vi "Get Output Values.vi"(6 "Last request":bool, 8 "error in (no error)":errorcluster, 10 "Number of points":i32, 11 "Spectrum Recorder in":refnum<class "Spectrum Recorder too.lvclass">) -> (0 "error out":errorcluster, 2 "Output values":dbl[](array[numeric]), 3 "Spectrum Recorder out":refnum<class "Spectrum Recorder too.lvclass">)   [LabVIEW 2016, in "Spectrum Recorder too.lvclass"]
uses:
  Spectrum Recorder too.lvclass
  C:/github/LabActor/Instrument Actor/Instrument Actor.lvclass
  Spectrum Recorder too.lvclass/Spectrum Recorder too.ctl
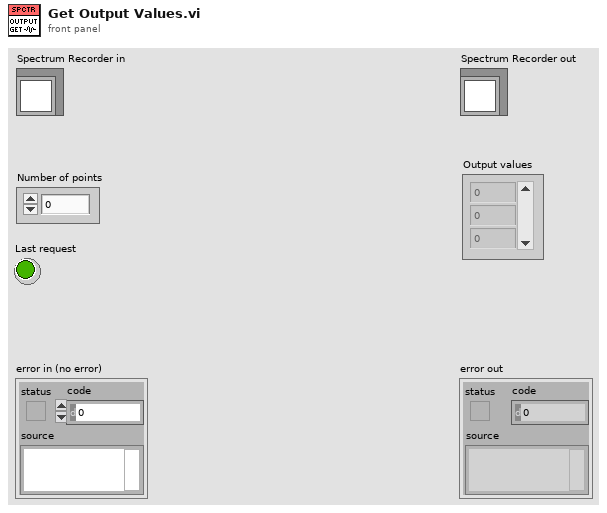
[diagram p1: front panel]
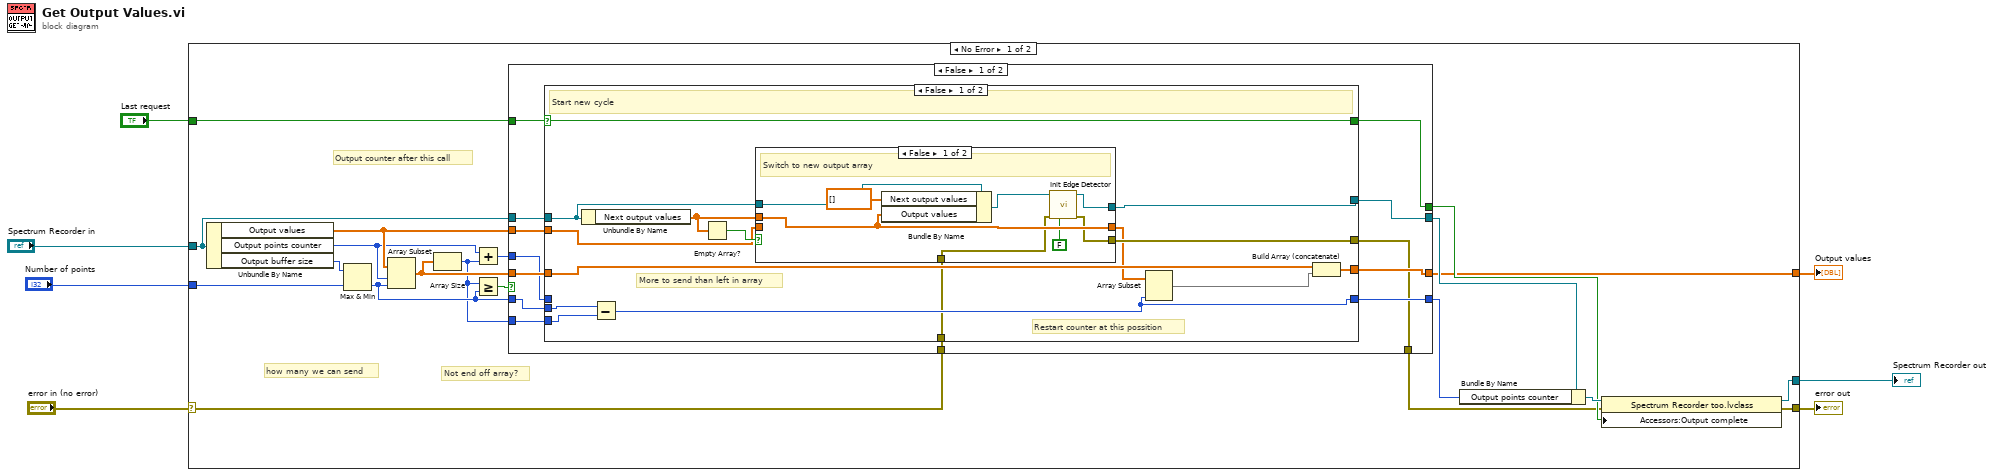
[diagram p0: block diagram]
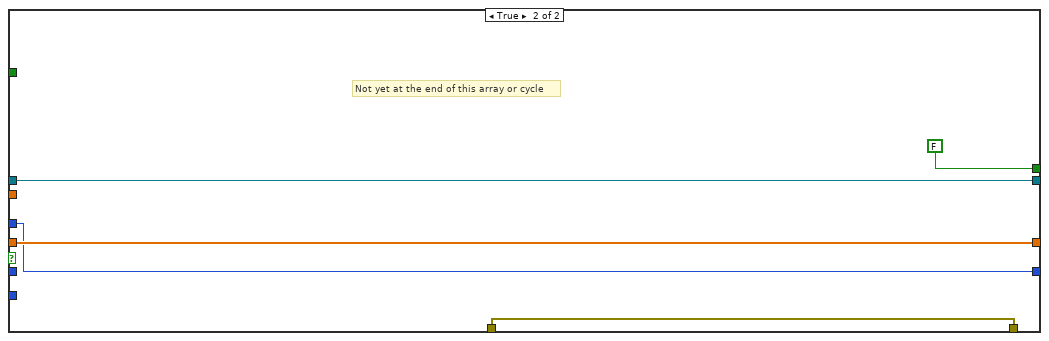
[diagram p4: hidden frame]
diagram:
  n1 = case shown="No Error" "error in (no error)" {
    selector: "error in (no error)" -> [w11 w78]
    tunnel: [w27 w78] -> w6
    tunnel: [w25 w77] -> w4
    tunnel: "Spectrum Recorder in" -> [w22 w77]
    tunnel: "Number of points" -> [w15 _]
    tunnel: [w10 _] -> w2
    tunnel: "Last request" -> [w23 _]
    frame No Error {
      # "Not end off array?"
      # "Output counter after this call"
      # "how many we can send"
      n2 = Unbundle By Name(w22) -> ("Output values"=w20:dbl[], "Output points counter"=w9:i32, "Output buffer size"=w14:i32)
      n3 = Max & Min(x=w14, y=w15) -> (min(x,y)=w21:i32)  [unwired: 1 out]
      n4 = Array Subset(array=w20, index=w9, length=w21) -> (w18:dbl[])
      n5 = Array Size(array=w18) -> (size(s)=w13:i32)
      n6 = Add(x=w9, y=w13) -> (x+y=w17:i32)
      n7 = Greater Or Equal?(x=w13, y=w21) -> (x >= y?=w24:bool)
      n8 = case shown="False" w24 {
        tunnel: w20 -> [w38 _]
        tunnel: w17 -> [w31 w74]
        tunnel: w21 -> [w28 _]
        tunnel: w23 -> [w40 _]
        tunnel: w22 -> [w39 w73]
        tunnel: [w36 w75] -> w10
        tunnel: w18 -> [w37 w75]
        tunnel: [w35 FALSE] -> w19
        tunnel: [w34 w74] -> w8
        tunnel: [w33 w73] -> w16
        tunnel: w13 -> [w32 _]
        tunnel: [w30 w72] -> w12
        tunnel: w11 -> [w29 w72]
        frame False {
          n9 = case shown="False" w40 {
            selector: w40 -> [w48 w71]
            tunnel: w39 -> [w54 w69]
            tunnel: w38 -> [w52 _]
            tunnel: w37 -> [w51 w68]
            tunnel: w31 -> [_ w70]
            tunnel: [w49 w68] -> w36
            tunnel: [w48 w71] -> w35
            tunnel: [w47 w70] -> w34
            tunnel: [w43 w69] -> w33
            tunnel: w32 -> [w46 _]
            tunnel: [w42 w67] -> w30
            tunnel: w29 -> [w45 w67]
            tunnel: w28 -> [w44 _]
            frame False {
              # "Restart counter at this possition"
              # "More to send than left in array"
              # "Start new cycle"
              n10 = Unbundle By Name(w54) -> ("Next output values"=w53:dbl[])
              n11 = Subtract(x=w44, y=w46) -> (x-y=w47:i32)
              n12 = Empty Array?(array=w53) -> (empty?=w55:bool)
              n13 = case shown="False" w55 {
                tunnel: w54 -> [w63 w66]
                tunnel: w53 -> [w62 _]
                tunnel: [w59 w66] -> w43
                tunnel: [w62 w65] -> w41
                tunnel: w52 -> [_ w65]
                tunnel: [w58 w64] -> w42
                tunnel: w45 -> [w57 w64]
                frame False {
                  # "Switch to new output array"
                  n14 = Bundle By Name(cluster=w63, "Next output values"=dbl[] [], "Output values"=w62) -> (w60:refnum<class "Spectrum Recorder too.lvclass">)
                  n15 = call-dynamic "Init Edge Detector.vi"("Unsee last word"=FALSE, "error in (no error)"=w57, "Spectrum Recorder too in"=w60) -> ("error out"=w58:errorcluster, "Spectrum Recorder too out"=w59:refnum<class "Spectrum Recorder too.lvclass">)  [unwired: 7 in]
                }
                frame True {
                  # "Repeat same output array"
                }
              }
              n16 = Array Subset(array=w41, length=w47) -> (w50:dbl[])  [unwired: 1 in]
              n17 = Build Array (concatenate)(w51, w50) -> (w49:dbl[])
            }
            frame True {
              # "All output done"
            }
          }
        }
        frame True {
          # "Not yet at the end of this array or cycle"
        }
      }
      n18 = Bundle By Name(cluster=w16, "Output points counter"=w8) -> (w26:refnum<class "Spectrum Recorder too.lvclass">)
      n19 = property class="Spectrum Recorder too.lvclass"(reference=w26, error in=w12, "Accessors:Output complete"=w19) -> (reference out=w25:refnum<class "Spectrum Recorder too.lvclass">, error out=w27:errorcluster)
    }
    frame Error {
    }
  }
  "error out" <- w6
  "Spectrum Recorder out" <- w4
  "Output values" <- w2
